vi "PTScanner.check add object.vi"(1 "Object cmds":T1[](array[typedef]), 4 "new obj command":T1, 5 "error in (no error)":errorcluster) -> (15 "Object cmds out":T1[](array[typedef]), 19 "error out":errorcluster)   [LabVIEW 2014, in "PTScanner.lvlib"]
uses:
  PTScanner.lvlib
  PTScanner.obj parameters.ctl
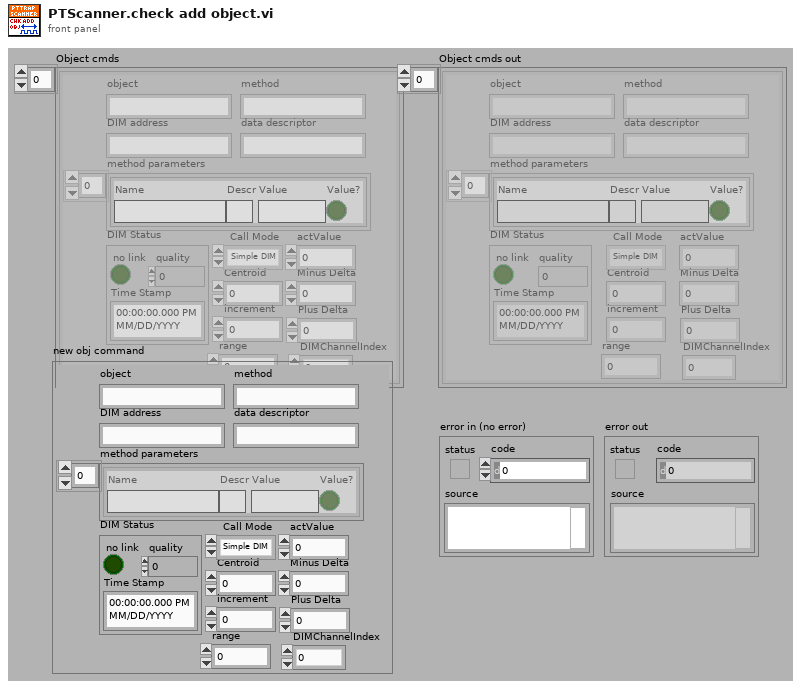
[diagram p1: front panel]
types:
  T1 = typedef "PTScanner.lvlib/PTScanner.obj parameters.ctl" = cluster{"object":string, "DIM address":string, "method":string, "data descriptor":string, "method parameters":cluster{"Name":string, "Descr":string, "Value":string, "Value?":bool}[], "Call Mode":enum16{"Simple DIM", "Synchronous"}, "actValue":dbl, "Centroid":dbl, "Minus Delta":dbl, "Plus Delta":dbl, "increment":dbl, "DIM Status":cluster{"no link":bool, "quality":i32, "Time Stamp":timestamp}, "range":dbl, "DIMChannelIndex":i32}
  T2 = cluster{"Name":string, "Descr":string, "Value":string, "Value?":bool}[]
  T3 = cluster{"object":string, "method":string, bool[], string[]}
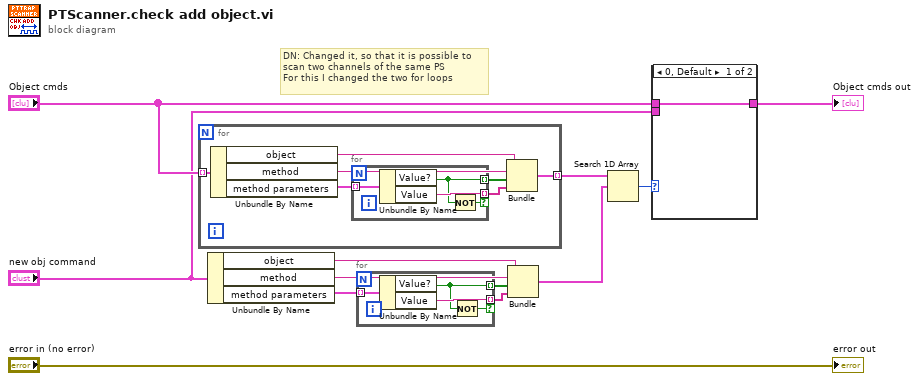
[diagram p0: block diagram]
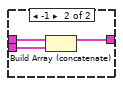
[diagram p2: hidden frame]
diagram:
  # "DN: Changed it, so that it is possible to\nscan two channels of the same PS\nFor this I changed the two for loops"
  n1 = for {
    tunnel: "Object cmds" -> [w19] mode=indexing
    tunnel: [w14] -> w4 mode=indexing
    n2 = Unbundle By Name(w19) -> ("object"=w17:string, "method"=w16:string, "method parameters"=w18:T2)
    n3 = for {
      tunnel: w18 -> [w23] mode=indexing
      tunnel: [w20] -> w15 mode=indexing
      tunnel: [w22] -> w13 mode=indexing if=w21
      n4 = Unbundle By Name(w23) -> ("Value?"=w20:bool, "Value"=w22:string)
      n5 = Not(x=w20) -> (.not. x?=w21:bool)
    }
    n6 = Bundle("object"=w17, "method"=w16, w15, w13) -> (w14:T3)  [unwired: 1 in]
  }
  n7 = Unbundle By Name("new obj command") -> ("object"=w7:string, "method"=w6:string, "method parameters"=w8:T2)
  n8 = for {
    tunnel: w8 -> [w27] mode=indexing
    tunnel: [w24] -> w5 mode=indexing
    tunnel: [w26] -> w1 mode=indexing if=w25
    n9 = Unbundle By Name(w27) -> ("Value?"=w24:bool, "Value"=w26:string)
    n10 = Not(x=w24) -> (.not. x?=w25:bool)
  }
  n11 = Bundle("object"=w7, "method"=w6, w5, w1) -> (w3:T3)  [unwired: 1 in]
  n12 = Search 1D Array(1D array=w4, element=w3) -> (index of element=w2:i32)  [unwired: 1 in]
  n13 = case shown="0, Default" w2 {
    tunnel: "Object cmds" -> [w28 w31]
    tunnel: [w28 w30] -> w10
    tunnel: "new obj command" -> [_ w29]
    frame 0, Default {
    }
    frame -1 {
      n14 = Build Array (concatenate)(w31, w29) -> (w30:T1[])
    }
  }
  "Object cmds out" <- w10
  "error out" <- "error in (no error)"
